vi "GFITS_WriteHeaders_quick.vi"(1 "Database RefNum in":T1, 5 "ref":u64, 7 "number of extensions":u16, 9 "Keywords":string[][][](array[string]), 11 "number of keywords":i32[](array[numeric]), 12 "expID in":string) -> (6 "ref out":u64, 8 "expID":string)   [LabVIEW 2016]
uses:
  DBSHAND/private/vis/DatabaseHand_RefNum.ctl
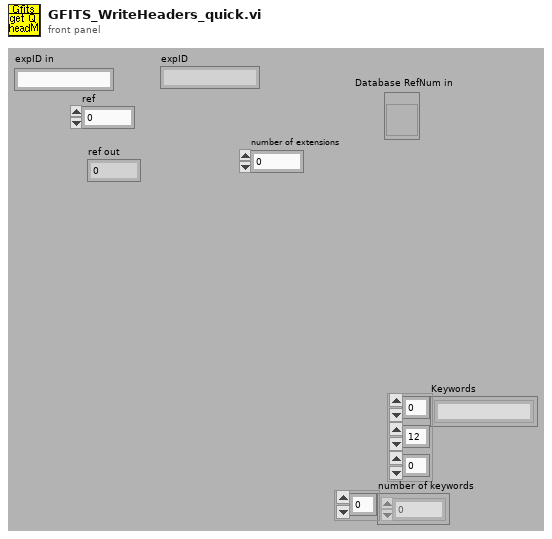
[diagram p1: front panel]
types:
  T1 = typedef "DatabaseHand_RefNum.ctl" = refnum<vi>
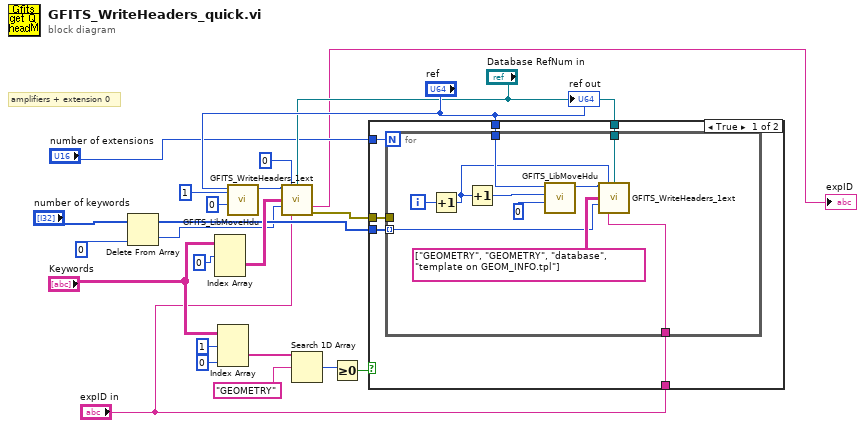
[diagram p0: block diagram]
diagram:
  # "amplifiers + extension 0"
  n1 = Delete From Array(array="number of keywords", index=0) -> (deleted portion=w10:i32, array with subset deleted=w11:i32[])  [unwired: 1 in]
  n2 = Index Array(array="Keywords", index (dim 0)=0 ("index (page)")) -> (element=w18:string[][])  [unwired: 2 in]
  n3 = Index Array(array="Keywords", index (dim 0)=1 ("index (page)"), index (dim 2)=0 ("disabled index (col)")) -> (element=w7:string[])  [unwired: 1 in]
  n4 = call "GFITS_LibMoveHdu.vi"("hdutype"=0, "hdunum"=1, "ref"="ref") -> ("ref out"=w23:u64)  [unwired: 1 in, 7 out]
  n5 = call "GFITS_WriteHeaders_1ext.vi"("ref"=w23, "extension"=0, "Database RefNum in"="Database RefNum in", "Keywords"=w18, "numer of keywords"=w10, "expID in"="expID in") -> ("expID"=→"expID":string, "error out"=w17:errorcluster)  [unwired: 1 in, 7 out]
  n6 = Search 1D Array(1D array=w7, element="GEOMETRY") -> (index of element=w5:i32)  [unwired: 1 out]
  n7 = Greater Or Equal To 0?(x=w5) -> (x >= 0?=w2:bool)
  n8 = case shown="True" w2 {
    tunnel: "ref" -> [w29 _]
    tunnel: "Database RefNum in" -> [w28 _]
    tunnel: w17 -> [w27 _]
    tunnel: "number of extensions" -> [w26 _]
    tunnel: w11 -> [w25 _]
    tunnel: "expID in" -> [w24 _]
    frame True {
      n9 = for {
        N: w26 -> [_]
        tunnel: w29 -> [w39]
        tunnel: w28 -> [w35]
        tunnel: w27 -> [_]
        tunnel: w25 -> [w31] mode=indexing
        tunnel: w24 -> [w30]
        i -> [w36]
        n10 = Increment(x=w36) -> (x+1=w33:i32)
        n11 = Increment(x=w33) -> (x+1=w34:i32)
        n12 = call "GFITS_LibMoveHdu.vi"("hdutype"=0, "hdunum"=w34, "ref"=w39) -> ("ref out"=w37:u64)  [unwired: 1 in, 7 out]
        n13 = call "GFITS_WriteHeaders_1ext.vi"("ref"=w37, "extension"=w33, "Database RefNum in"=w35, "Keywords"=string[][] [["GEOMETRY", "GEOMETRY", "database", "template on GEOM_INFO.tpl"]], "numer of keywords"=w31, "expID in"=w30) -> ()  [unwired: 1 in, 9 out]
      }
    }
    frame False {
    }
  }
  "ref out" <- "ref"
